vi "Sample Group Data.vi"(7 "Buffer Used in":u32, 8 "error in (no error)":errorcluster, 9 "Data FIFO Buffer in":dbl[](array[numeric]), 10 "Data FIFO in":refnum<k33>, 11 "Group Sample Spec in":T1 {"Decimation Ref" format="%.0x"; "Block Refs"."Data Reference" format="%.0x"}) -> (0 "error out":errorcluster, 1 "Data FIFO Buffer out":dbl[](array[numeric]), 2 "Data FIFO out":refnum<k33>, 3 "Group Sample Spec out":T1 {"Decimation Ref" format="%.0x"; "Block Refs"."Data Reference" format="%.0x"}, 4 "Timeout":bool, 5 "Buffer Used out":u32)   [LabVIEW 2027, in "Embedded Data Logger Engine.lvlib"]
uses:
  Embedded Data Logger Engine.lvlib
  Group Sampling Specification.ctl
  <vilib>/NI VeriStand/Custom Device API/Block Data Reference.ctl
  <vilib>/NI VeriStand/Custom Device API/Data Reference.ctl
  <vilib>/NI VeriStand/Custom Device API/Global Data Refs.vi
  <vilib>/NI VeriStand/Custom Device API/Custom Device API.lvlib
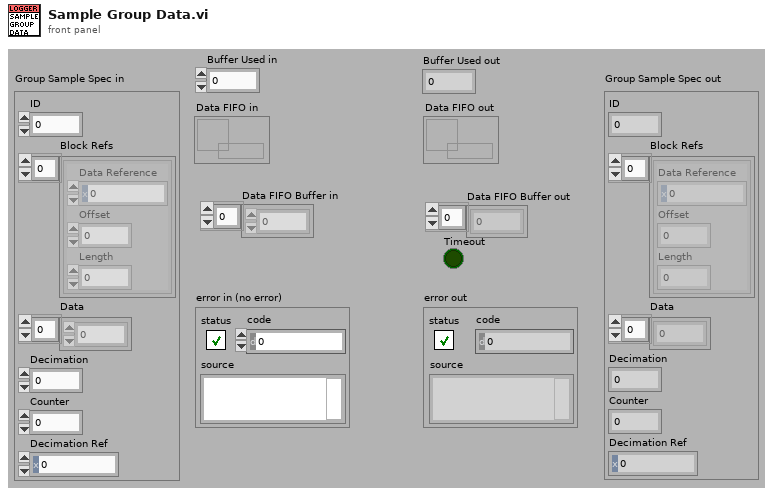
[diagram p1: front panel]
types:
  T1 = typedef "Embedded Data Logger Engine.lvlib/Group Sampling Specification.ctl" = cluster{"ID":dbl, "Block Refs":T2[], "Data":dbl[], "Decimation":i32, "Counter":i32, "Decimation Ref":T3}
  T2 = typedef "Custom Device API.lvlib/Block Data Reference.ctl" = cluster{"Data Reference":T3, "Offset":u64, "Length":u64}
  T3 = typedef "Custom Device API.lvlib/Data Reference.ctl" = i32
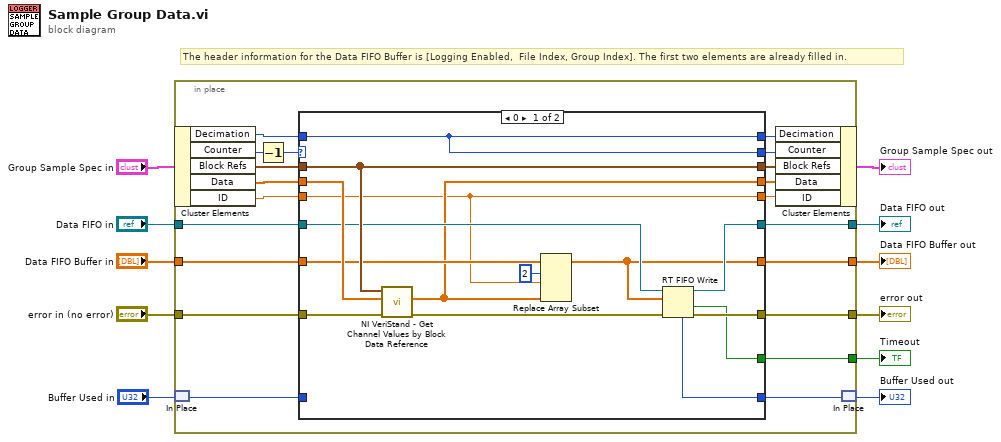
[diagram p0: block diagram]
diagram:
  # "The header information for the Data FIFO Buffer is [Logging Enabled,  File Index, Group Index]. The first two elements are already filled in."
  n1 = in-place {
    in-place-border: "error in (no error)" -> [w22]
    in-place-border: [w21] -> w11
    in-place-border: "Data FIFO in" -> [w20]
    in-place-border: "Data FIFO Buffer in" -> [w17]
    in-place-border: [w19] -> w5
    in-place-border: [w18] -> w4
    in-place-border: [w14] -> w3
    n2 = in-place-cluster #1("Group Sample Spec in") -> ("Decimation"=w29:i32, "Counter"=w31:i32, "Block Refs"=w26:T2[], "Data"=w23:dbl[], "ID"=w16:dbl)
    n3 = in-place-match #2("Buffer Used in") -> (w13:u32)
    n4 = Decrement(x=w31) -> (x-1=w30:i32)
    n5 = case shown="0" w30 {
      selector: w30 -> [_ w54]
      tunnel: w29 -> [w45 w55]
      tunnel: [w45 w55] -> w28
      tunnel: [w45 w54] -> w27
      tunnel: w26 -> [w43 w53]
      tunnel: [w43 w53] -> w25
      tunnel: [w37 w52] -> w24
      tunnel: w23 -> [w44 w52]
      tunnel: w22 -> [w46 w51]
      tunnel: [w39 w51] -> w21
      tunnel: w20 -> [w41 w50]
      tunnel: [w40 w50] -> w19
      tunnel: [w36 w49] -> w18
      tunnel: w17 -> [w38 w49]
      tunnel: w16 -> [w35 w48]
      tunnel: [w35 w48] -> w15
      tunnel: [w33 w47] -> w12
      tunnel: [w32 _] -> w14
      tunnel: w13 -> [_ w47]
      frame 0 {
        n6 = call <vilib>:"NI VeriStand - Get Channel Values by Block Data Reference.vi"("error in (no error)"=w46, "Values Array in"=w44, "Block Data Ref"=w43) -> ("error out"=w42:errorcluster, "Values Array out"=w37:dbl[])  [unwired: 7 out]
        n7 = Replace Array Subset(array=w38, new element #1=w35, index #1=2 ("index"), new element #2=w37) -> (w36:dbl[])  [unwired: 1 in]
        n8 = RT FIFO Write(0:w41, 1:w36, 3:w42) -> (7:w33:u32, 8:w40:refnum<k33>, 10:w32:bool, 11:w39:errorcluster)  [unwired: 1 in, 1 out]
      }
      frame Default {
      }
    }
    n9 = in-place-cluster #1("Decimation"=w28, "Counter"=w27, "Block Refs"=w25, "Data"=w24, "ID"=w15) -> (→"Group Sample Spec out":T1)
    n10 = in-place-match #2(w12) -> (→"Buffer Used out":u32)
  }
  "error out" <- w11
  "Data FIFO out" <- w5
  "Data FIFO Buffer out" <- w4
  "Timeout" <- w3
